vi "license file.vi"(1 "year":u16=2005) -> (0 "Accepted":bool)   [LabVIEW 2015]
uses:
  Process Controller 3.0/Calibration and Function folders.ctl
  <vilib>/Utility/config.llb/Read Key (Boolean).vi
  <vilib>/Utility/config.llb/Write Key (Boolean).vi
  <vilib>/Utility/config.llb/NI_LVConfig.lvlib
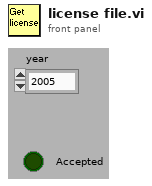
[diagram p1: front panel]
types:
  T1 = typedef "Calibration and Function folders.ctl" = enum16{"Sensors", "Functions", "Config File", "PublicAppFolder", "New ini File", "Set Config File", "Delete ini File"}
  T2 = typedef "NI_LVConfig.lvlib/Config Data RefNum.ctl" = refnum<k1>
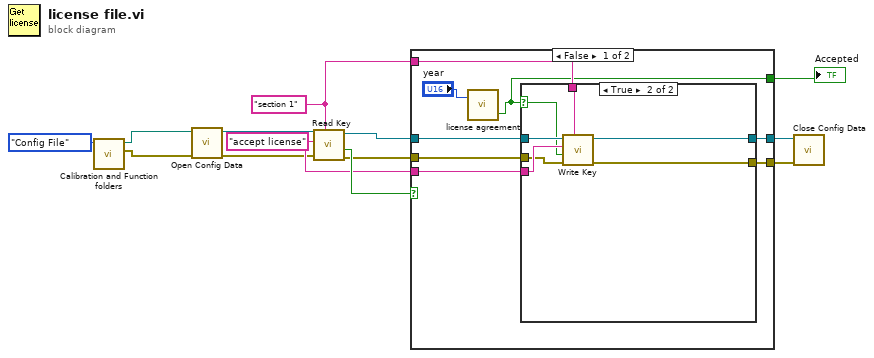
[diagram p0: block diagram]
diagram:
  w9 = "section 1" ("section")
  w10 = "accept license" ("key")
  n1 = call "Calibration and Function folders.vi"("Folder"=Calibration_and_Function_folders."Config File") -> ("error out"=w2:errorcluster, "Selected Folder"=w4:path)  [unwired: 9 in]
  n2 = call <vilib>:"Open Config Data.vi"("error in (no error)"=w2, "configuration file path"=w4) -> ("error out"=w1:errorcluster, "refnum"=w13:T2)  [unwired: 7 in, 1 out]
  n3 = call-poly <vilib>:"Read Key.vi"("section"=w9, "error in (no error)"=w1, "key"=w10, "refnum"=w13) -> ("error out"=w6:errorcluster, "value"=w12:bool, "refnum out"=w11:T2)  [unwired: 4 in, 1 out]
  n4 = case shown="False" w12 {
    selector: w12 -> [_ w31]
    tunnel: w11 -> [w20 w33]
    tunnel: w10 -> [w19 _]
    tunnel: w9 -> [w18 _]
    tunnel: [w17 w33] -> w8
    tunnel: [w16 w32] -> w7
    tunnel: w6 -> [w15 w32]
    tunnel: [w14 w31] -> w5
    frame False {
      n5 = call "license agreement.vi"("year"="year") -> ("Accepted"=w14:bool)  [unwired: 1 in, 1 out]
      n6 = case shown="True" w14 {
        selector: w14 -> [_ w28]
        tunnel: w20 -> [w23 w30]
        tunnel: w19 -> [_ w29]
        tunnel: w18 -> [_ w27]
        tunnel: [w23 w26] -> w17
        tunnel: [w22 w25] -> w16
        tunnel: w15 -> [w22 w24]
        frame False {
        }
        frame True {
          n7 = call-poly <vilib>:"Write Key.vi"("section"=w27, "error in (no error)"=w24, "value"=w28, "key"=w29, "refnum"=w30) -> ("error out"=w25:errorcluster, "refnum out"=w26:T2)  [unwired: 4 in, 1 out]
        }
      }
    }
    frame True {
    }
  }
  "Accepted" <- w5
  n8 = call <vilib>:"Close Config Data.vi"("error in (no error)"=w7, "refnum"=w8) -> ()  [unwired: 8 in, 2 out]
